vi "ReadIEEE BlockR4.vi"(8 "error in (no error)":errorcluster {"code" format="%.0x"}, 9 "ValBufferSize":i32=2048, 11 "instrument handle":refnum<k15>) -> (0 "error out":errorcluster {"code" format="%.0x"}, 1 "ValActualSize":i32, 2 "Val":sgl[](array[numeric]), 3 "instrument handle out":refnum<k15>)   [LabVIEW 2014, in "Agilent NA.lvlib"]
doc: "Read definite-length IEEE binary block the I/O stream"
uses:
  Agilent NA.lvlib
  AgNA.dll
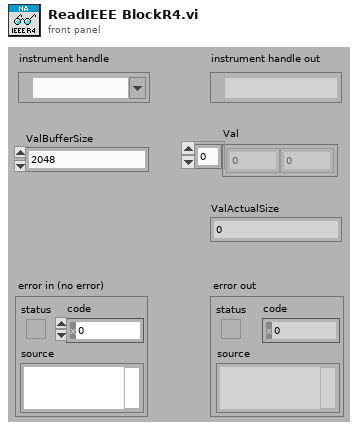
[diagram p1: front panel]
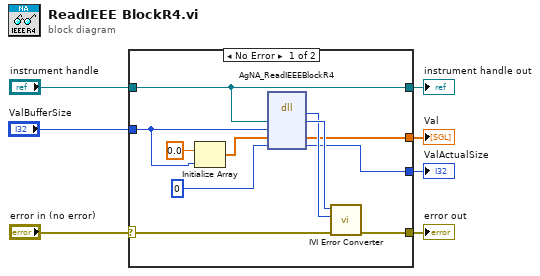
[diagram p0: block diagram]
diagram:
  n1 = case shown="No Error" "error in (no error)" {
    selector: "error in (no error)" -> [w16 w20]
    tunnel: [w15 w20] -> w7
    tunnel: "ValBufferSize" -> [w8 _]
    tunnel: [w14 _] -> w1
    tunnel: [w13 _] -> w4
    tunnel: [w12 w19] -> w3
    tunnel: "instrument handle" -> [w12 w19]
    frame No Error {
      n2 = Initialize Array(sgl 0.0 ("element"), w8) -> (w9:sgl[])
      n3 = dll-call lib="AgNA**.dll" fn="AgNA_ReadIEEEBlockR4"("Vi"=w12, "ValBufferSize"=w8, "Val"=w9, "ValActualSize"=0) -> ("return type"=w17:i32, "Vi"=w18:u32, "Val"=w14:sgl[], "ValActualSize"=w13:i32)  [unwired: 4 in, 2 out]
      n4 = call "IVI Error Converter.vi"("error in (no error)"=w16, "IVI error code (0)"=w17, "instrument handle"=w18) -> ("error out"=w15:errorcluster)  [unwired: 7 in, 1 out]
    }
    frame Error {
    }
  }
  "error out" <- w7
  "instrument handle out" <- w3
  "ValActualSize" <- w4
  "Val" <- w1
